vi "Size Column Width to Text.vi"(8 "error in":errorcluster, 11 "MulticolumnListbox":refnum<vi>) -> (0 "error out":errorcluster)   [LabVIEW 2017, in "Message Log.lvclass"]
uses:
  Message Log.lvclass
  <vilib>/Utility/miscctls.llb/LVRowAndColumnTypeDef.ctl
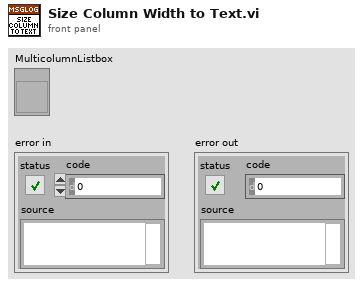
[diagram p1: front panel]
types:
  T1 = typedef "LVRowAndColumnTypeDef.ctl" = cluster{"Row":i32, "Column":i32}
  T2 = cluster{"left":i16, "top":i16, "right":i16, "bottom":i16}
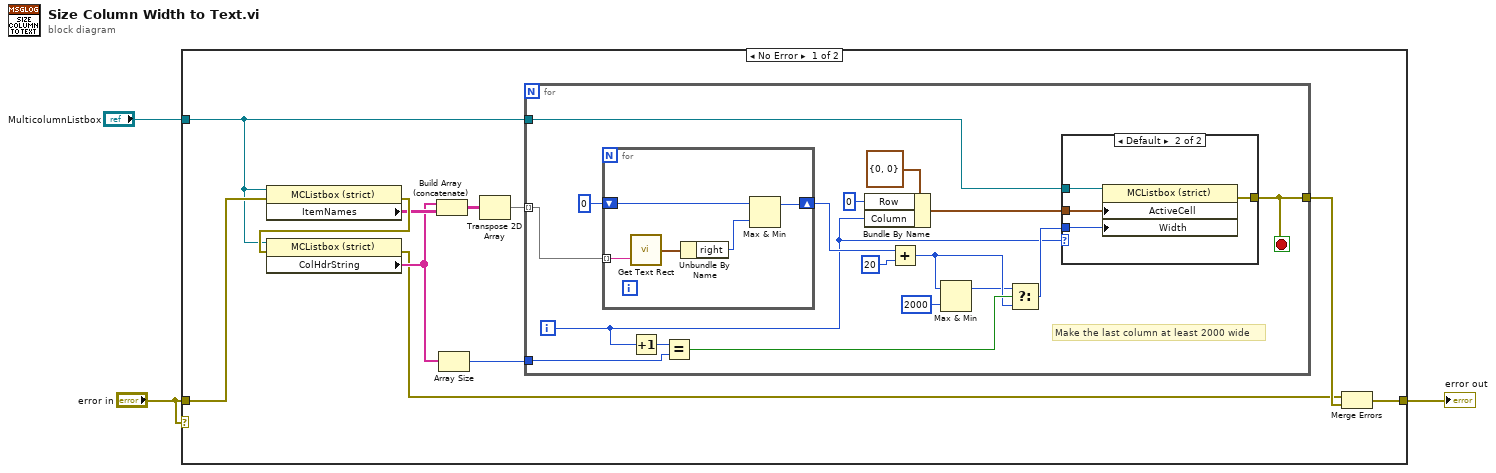
[diagram p0: block diagram]
diagram:
  n1 = case shown="No Error" "error in" {
    tunnel: "MulticolumnListbox" -> [w6 _]
    tunnel: [w13 w41] -> w2
    tunnel: "error in" -> [w11 w41]
    frame No Error {
      n2 = property class="MCListbox (strict)"(reference=w6, error in=w11) -> (error out=w14:errorcluster, "ItemNames"=w10:string[][])  [unwired: 1 out]
      n3 = property class="MCListbox (strict)"(reference=w6, error in=w14) -> (error out=w5:errorcluster, "ColHdrString"=w7:string[])  [unwired: 1 out]
      n4 = Build Array (concatenate)(w7, w10) -> (w9:string[][])
      n5 = Array Size(array=w7) -> (size(s)=w4:i32)
      n6 = Transpose 2D Array(2D array=w9) -> (transposed array=w8:string[][])
      n7 = for {
        tunnel: [w31] -> w12
        tunnel: w6 -> [w30]
        tunnel: w8 -> [w29] mode=indexing
        tunnel: w4 -> [w21]
        i -> [w15]
        stop <- w31 stop-if-true
        # "Make the last column at least 2000 wide"
        n8 = for {
          shift-right: [w38] -> w23
          shift-left: 0 -> [w39]
          tunnel: w29 -> [w36] mode=indexing
          n9 = call <vilib>:"Get Text Rect.vi"("text"=w36) -> ("rect"=w40:T2)  [unwired: 8 in]
          n10 = Unbundle By Name(w40) -> ("right"=w37:i16)
          n11 = Max & Min(x=w39, y=w37) -> (max(x,y)=w38:i32)  [unwired: 1 out]
        }
        n12 = Increment(x=w15) -> (x+1=w22:i32)
        n13 = Equal?(x=w22, y=w21) -> (x = y?=w20:bool)
        n14 = Bundle By Name(cluster=T1 {"Row"=0, "Column"=0} ("Active Cell:Active Cell"), "Row"=0, "Column"=w15) -> (w25:T1)
        n15 = Add(x=w23, y=20) -> (x+y=w18:i32)
        n16 = Max & Min(x=w18, y=2000) -> (max(x,y)=w17:i32)  [unwired: 1 out]
        n17 = Select(t=w17, s=w20, f=w18) -> (s? t:f=w19:i32)
        n18 = case shown="Default" w15 {
          tunnel: [_ w35] -> w31
          tunnel: w30 -> [_ w34]
          tunnel: w25 -> [_ w33]
          tunnel: w19 -> [_ w32]
          frame 0 {
            # "First column\nnever auto size"
          }
          frame Default {
            n19 = property class="MCListbox (strict)"(reference=w34, "ActiveCell"=w33, "Width"=w32) -> (error out=w35:errorcluster)  [unwired: 1 in, 1 out]
          }
        }
      }
      n20 = Merge Errors(w5, w12) -> (w13:errorcluster)
    }
    frame Error {
    }
  }
  "error out" <- w2
